vi "CTR_webSocketConfig_XML-JSON.vi"(8 "error in":errorcluster, 10 "webSocketCluster_typeDef in":T2, 11 "DOM document in":refnum<k20>) -> (0 "error out":errorcluster={"status"=TRUE, "code"=0, "source"=""}, 2 "webSocketCluster_typeDef out":T2, 3 "DOM document out":refnum<k20>)   [LabVIEW 2024]
uses:
  10f0a1c7-9ed0-4649-ba5a-dd6b15093da3.vi
  0a0fd023-9856-4cf8-bcff-a165bffb7d59.vi
  <vilib>/xml/Close Reference(Node).vi
  <vilib>/Utility/error.llb/Error Cluster From Error Code.vi
  <vilib>/ErrorRing/Error Ring.xnode
  <vilib>/Comparison/Less/Less Functor/Less Functor.lvclass
  <vilib>/xml/NI_XML.lvlib
  Control/webSocketCluster_typeDef.ctl
  Control/webSocketJsonConfig.ctl
panel:
  in  "webSocketJsonConfig":T1={"controls"=[{"channels"=[{"refDes"="OT-01", "role"="sensor", "units"="Deg F"}], "type"="temperature", "description"="LOX Tank Temperature 0%", "refDes"="OT-01", "subType"="", "details"={"absolute"=FALSE, "absoluteSensorRefDes"="NPT-01", "senseRefDes"="NPT-02"}}], "type"="config"}
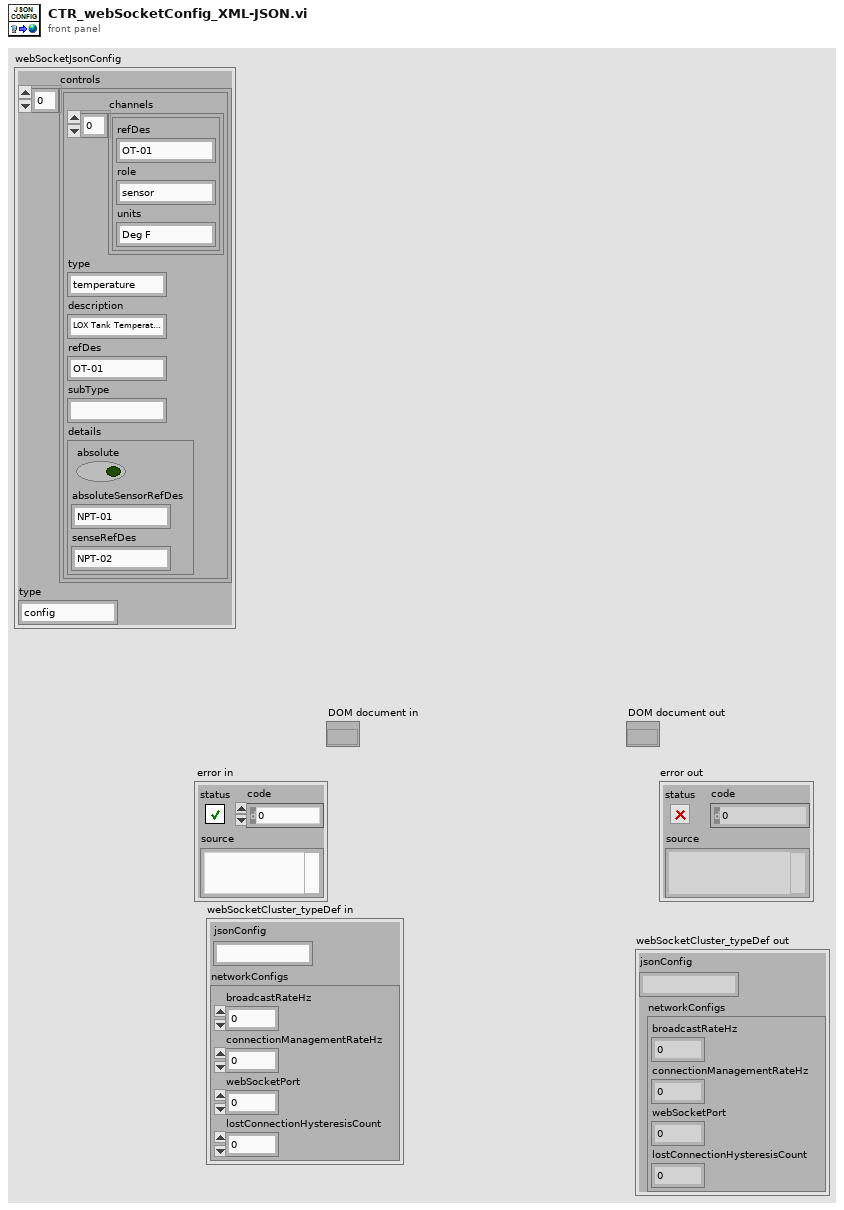
[diagram p1: front panel]
types:
  T1 = typedef "webSocketJsonConfig.ctl" = cluster{"controls":cluster{"channels":cluster{"refDes":string, "role":string, "units":string}[], "type":string, "description":string, "refDes":string, "subType":string, "details":cluster{"absolute":bool, "absoluteSensorRefDes":string, "senseRefDes":string}}[], "type":string}
  T2 = typedef "webSocketCluster_typeDef.ctl" = cluster{"networkConfigs":cluster{"broadcastRateHz":i32, "connectionManagementRateHz":i32, "webSocketPort":i32, "lostConnectionHysteresisCount":i32}, "jsonConfig":string}
  T3 = cluster{"channels":cluster{"refDes":string, "role":string, "units":string}[], "type":string, "description":string, "refDes":string, "subType":string, "details":cluster{"absolute":bool, "absoluteSensorRefDes":string, "senseRefDes":string}}[]
  T4 = cluster{"refDes":string, "role":string, "units":string}[]
  T5 = cluster{"absolute":bool, "absoluteSensorRefDes":string, "senseRefDes":string}
  T6 = cluster{"[0]":string, "[1]":string, "[2]":string}
  T7 = cluster{"refDes":string, "role":string, "units":string}
  T8 = cluster{"[0]":string, "[1]":string, "[2]":string, "[3]":string}
  T9 = cluster{"channels":cluster{"refDes":string, "role":string, "units":string}[], "type":string, "description":string, "refDes":string, "subType":string, "details":cluster{"absolute":bool, "absoluteSensorRefDes":string, "senseRefDes":string}}
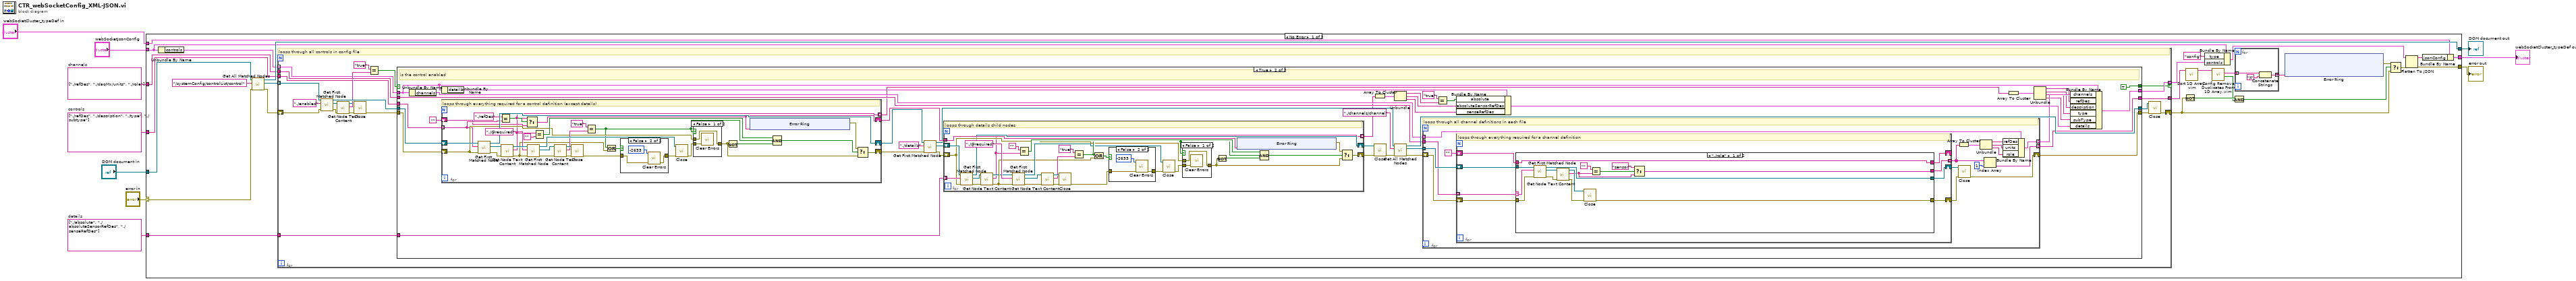
[diagram p0: block diagram]
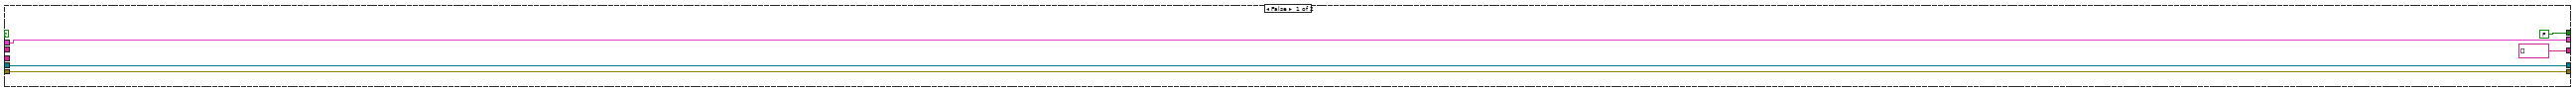
[diagram p2: hidden frame]
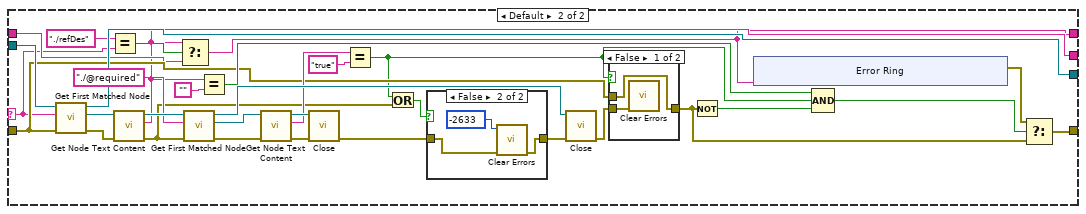
[diagram p7: hidden frame]
diagram:
  w1 = string[] ["./absolute", "./absoluteSensorRefDes", "./senseRefDes"]  # details
  w2 = string[] ["./refDes", "./description", "./type", "./subtype"]  # controls
  w7 = string[] ["./refDes", "./daqMx/units", "./role"]  # channels
  n1 = case shown="No Error" "error in" {
    selector: "error in" -> [w37 w297]
    tunnel: [w18 w297] -> w9
    tunnel: [w33 w296] -> w8
    tunnel: "DOM document in" -> [w38 w296]
    tunnel: w7 -> [w32 _]
    tunnel: "webSocketCluster_typeDef in" -> [w22 w295]
    tunnel: [w21 w295] -> w4
    tunnel: "webSocketJsonConfig" -> [w14 _]
    tunnel: w2 -> [w12 _]
    tunnel: w1 -> [w11 _]
    frame No Error {
      n2 = Unbundle By Name(w14) -> ("controls"=w13:T3)
      n3 = call <vilib>:"Get All Matched Nodes.vi"("error in (no error)"=w37, "XPath expression"="/systemConfig/controlList/control", "node in"=w38) -> ("error out"=w34:errorcluster, "node result array"=w35:refnum<k20>[], "node out"=w33:refnum<k20>)  [unwired: 6 in]
      n4 = for {
        tunnel: w35 -> [w61] mode=indexing
        shift-right: [w68] -> w28
        shift-left: w34 -> [w64]
        tunnel: w32 -> [w67]
        tunnel: [w54] -> w31 mode=concatenating
        tunnel: [w53] -> w17 mode=indexing if=w51
        tunnel: w13 -> [w52] mode=indexing
        tunnel: w12 -> [w50]
        tunnel: w11 -> [w49]
        # "loops through all controls in config file"
        n5 = call <vilib>:"Get First Matched Node.vi"("error in (no error)"=w64, "XPath expression"="./enabled", "node in"=w61) -> ("error out"=w65:errorcluster, "node result"=w59:refnum<k20>, "node out"=w62:refnum<k20>)  [unwired: 6 in]
        n6 = call <vilib>:"Get Node Text Content.vi"("error in (no error)"=w65, "node in"=w59) -> ("error out"=w66:errorcluster, "node text"=w57:string, "node out"=w56:refnum<k20>)  [unwired: 7 in]
        n7 = call-poly <vilib>:"Close.vi"("error in (no error)"=w66, "node"=w56) -> ("error out"=w63:errorcluster)  [unwired: 7 in]
        n8 = Equal?(x="true", y=w57) -> (x = y?=w58:bool)
        n9 = case shown="True" w58 {
          tunnel: w63 -> [w74 w106]
          tunnel: w62 -> [w75 w105]
          tunnel: [w74 w114] -> w70
          tunnel: [w75 w113] -> w69
          tunnel: w67 -> [_ w103]
          tunnel: [string[] [] w112] -> w54
          tunnel: [w71 w111] -> w53
          tunnel: w52 -> [w71 w85]
          tunnel: [FALSE TRUE] -> w51
          tunnel: w50 -> [_ w104]
          tunnel: w49 -> [_ w96]
          frame False {
          }
          frame True {
            # "is the control enabled"
            n10 = Unbundle By Name(w85) -> ("channels"=w108:T4)
            n11 = Unbundle By Name(w85) -> ("details"=w84:T5)
            n12 = for {
              shift-right: [w191] -> w91
              shift-left: w105 -> [w194]
              tunnel: w104 -> [w166] mode=indexing
              shift-right: [w176] -> w94
              shift-left: w106 -> [w172]
              tunnel: [w163] -> w102 mode=indexing
              shift-right: [w162] -> w95
              shift-left: "" -> [w164]
              # "loops through everything required for a control definition (except details)"
              n13 = call <vilib>:"Get First Matched Node.vi"("error in (no error)"=w172, "XPath expression"=w166, "node in"=w194) -> ("error out"=w193:errorcluster, "node result"=w192:refnum<k20>, "node out"=w191:refnum<k20>)  [unwired: 6 in]
              n14 = Equal?(x="./refDes", y=w166) -> (x = y?=w165:bool)
              n15 = call <vilib>:"Get Node Text Content.vi"("error in (no error)"=w193, "node in"=w192) -> ("error out"=w168:errorcluster, "node text"=w163:string, "node out"=w190:refnum<k20>)  [unwired: 7 in]
              n16 = Select(t=w163, s=w165, f=w164) -> (s? t:f=w162:string)
              n17 = call <vilib>:"Get First Matched Node.vi"("error in (no error)"=w168, "XPath expression"="./@required" ("string"), "node in"=w190) -> ("error out"=w189:errorcluster, "node result"=w188:refnum<k20>, "node out"=w187:refnum<k20>)  [unwired: 6 in]
              n18 = Equal?(x=w163, y="") -> (x = y?=w180:bool)
              n19 = call <vilib>:"Get Node Text Content.vi"("error in (no error)"=w189, "node in"=w188) -> ("error out"=w186:errorcluster, "node text"=w183:string, "node out"=w185:refnum<k20>)  [unwired: 7 in]
              n20 = call-poly <vilib>:"Close.vi"("error in (no error)"=w186, "node"=w185) -> ("error out"=w174:errorcluster)  [unwired: 7 in]
              n21 = Equal?(x="true" ("y"), y=w183) -> (x = y?=w169:bool)
              n22 = Or(x=w169, y=w168) -> (x .or. y?=w170:bool)
              n23 = case shown="False" w170 {
                tunnel: [w198 w200] -> w175
                tunnel: w174 -> [w198 w199]
                frame True {
                }
                frame False {
                  n24 = call <vilib>:"Clear Errors.vi"("error in (no error)"=w199, "specific error code to clear (0: all)"=-2633) -> ("error out"=w200:errorcluster)  [unwired: 4 in, 1 out]
                }
              }
              n25 = call-poly <vilib>:"Close.vi"("error in (no error)"=w175, "node"=w187) -> ("error out"=w173:errorcluster)  [unwired: 7 in]
              n26 = case shown="False" w169 {
                tunnel: w173 -> [w196 w197]
                tunnel: w172 -> [w195 _]
                tunnel: [w195 w197] -> w171
                frame False {
                  n27 = call <vilib>:"Clear Errors.vi"("error in (no error)"=w196) -> ()  [unwired: 5 in, 2 out]
                }
                frame True {
                }
              }
              n28 = Not(x=w171) -> (.not. x?=w179:bool)
              n29 = xnode "Error Ring"("parameter 0"=w162) -> ("error out"=w177:errorcluster)
              n30 = Compound Arithmetic op=AND(w180, w169, w179) -> (w178:bool)
              n31 = Select(t=w177, s=w178, f=w171) -> (s? t:f=w176:errorcluster)
            }
            n32 = call <vilib>:"Get First Matched Node.vi"("error in (no error)"=w94, "XPath expression"="./details", "node in"=w91) -> ("error out"=w93:errorcluster, "node result"=w89:refnum<k20>, "node out"=w90:refnum<k20>)  [unwired: 6 in]
            n33 = for {
              shift-right: [w144] -> w88
              shift-left: w93 -> [w122]
              tunnel: w96 -> [w123] mode=indexing
              tunnel: w95 -> [w143]
              shift-right: [w120] -> w87
              shift-left: w89 -> [w124]
              tunnel: [w118] -> w81 mode=indexing
              # "loops through details child nodes"
              n34 = call <vilib>:"Get First Matched Node.vi"("error in (no error)"=w122, "XPath expression"=w123, "node in"=w124) -> ("error out"=w125:errorcluster, "node result"=w126:refnum<k20>, "node out"=w120:refnum<k20>)  [unwired: 6 in]
              n35 = call <vilib>:"Get Node Text Content.vi"("error in (no error)"=w125, "node in"=w126) -> ("error out"=w121:errorcluster, "node text"=w118:string, "node out"=w119:refnum<k20>)  [unwired: 7 in]
              n36 = call <vilib>:"Get First Matched Node.vi"("error in (no error)"=w121, "XPath expression"="./@required" ("string"), "node in"=w119) -> ("error out"=w134:errorcluster, "node result"=w133:refnum<k20>, "node out"=w129:refnum<k20>)  [unwired: 6 in]
              n37 = Equal?(x="", y=w118) -> (x = y?=w138:bool)
              n38 = call <vilib>:"Get Node Text Content.vi"("error in (no error)"=w134, "node in"=w133) -> ("error out"=w132:errorcluster, "node text"=w128:string, "node out"=w131:refnum<k20>)  [unwired: 7 in]
              n39 = call-poly <vilib>:"Close.vi"("error in (no error)"=w132, "node"=w131) -> ("error out"=w130:errorcluster)  [unwired: 7 in]
              n40 = Equal?(x="true", y=w128) -> (x = y?=w135:bool)
              n41 = Or(x=w135, y=w121) -> (x .or. y?=w140:bool)
              n42 = case shown="False" w140 {
                tunnel: [w151 w153] -> w142
                tunnel: w130 -> [w151 w152]
                frame True {
                }
                frame False {
                  n43 = call <vilib>:"Clear Errors.vi"("error in (no error)"=w152, "specific error code to clear (0: all)"=-2633) -> ("error out"=w153:errorcluster)  [unwired: 4 in, 1 out]
                }
              }
              n44 = call-poly <vilib>:"Close.vi"("error in (no error)"=w142, "node"=w129) -> ("error out"=w141:errorcluster)  [unwired: 7 in]
              n45 = case shown="False" w135 {
                tunnel: w141 -> [w149 w150]
                tunnel: w122 -> [w148 _]
                tunnel: [w148 w150] -> w139
                frame False {
                  n46 = call <vilib>:"Clear Errors.vi"("error in (no error)"=w149) -> ()  [unwired: 5 in, 2 out]
                }
                frame True {
                }
              }
              n47 = Not(x=w139) -> (.not. x?=w145:bool)
              n48 = xnode "Error Ring"("parameter 0"=w143) -> ("error out"=w147:errorcluster)
              n49 = Compound Arithmetic op=AND(w138, w135, w145) -> (w146:bool)
              n50 = Select(t=w147, s=w146, f=w139) -> (s? t:f=w144:errorcluster)
            }
            n51 = Array To Cluster(array=w81) -> (cluster=w82:T6)
            n52 = call-poly <vilib>:"Close.vi"("error in (no error)"=w88, "node"=w87) -> ("error out"=w86:errorcluster)  [unwired: 7 in]
            n53 = Unbundle(w82) -> ("[0]"=w78:string, "[1]"=w79:string, "[2]"=w80:string)
            n54 = call <vilib>:"Get All Matched Nodes.vi"("error in (no error)"=w86, "XPath expression"="./channels/channel", "node in"=w90) -> ("error out"=w116:errorcluster, "node result array"=w115:refnum<k20>[], "node out"=w113:refnum<k20>)  [unwired: 6 in]
            n55 = for {
              shift-right: [w222] -> w114
              shift-left: w116 -> [w223]
              tunnel: w115 -> [w224] mode=indexing
              tunnel: w103 -> [w221]
              tunnel: [w218] -> w112 mode=indexing
              tunnel: [w216] -> w109 mode=indexing
              tunnel: w108 -> [w217] mode=indexing
              # "loops through all channel definitions in each file"
              n56 = for {
                shift-right: [w231] -> w215
                shift-left: w224 -> [w232]
                tunnel: w221 -> [w225] mode=indexing
                shift-right: [w230] -> w214
                shift-left: w223 -> [w229]
                tunnel: [w227] -> w212 mode=indexing
                shift-right: [w226] -> _
                shift-left: "" -> [w228]
                # "loops through everything required for a channel definition"
                n57 = case shown="\"./role\"" w225 {
                  selector: w225 -> [w243 w248]
                  tunnel: w232 -> [w242 w280]
                  tunnel: [w241 w277] -> w231
                  tunnel: [w238 w262] -> w230
                  tunnel: w229 -> [w244 w258]
                  tunnel: w228 -> [w247 w251]
                  tunnel: [w233 w250] -> w227
                  tunnel: [w247 w249] -> w226
                  frame "./role" {
                    n58 = call <vilib>:"Get First Matched Node.vi"("error in (no error)"=w244, "XPath expression"=w243, "node in"=w242) -> ("error out"=w246:errorcluster, "node result"=w240:refnum<k20>, "node out"=w241:refnum<k20>)  [unwired: 6 in]
                    n59 = call <vilib>:"Get Node Text Content.vi"("error in (no error)"=w246, "node in"=w240) -> ("error out"=w245:errorcluster, "node text"=w234:string, "node out"=w239:refnum<k20>)  [unwired: 7 in]
                    n60 = call-poly <vilib>:"Close.vi"("error in (no error)"=w245, "node"=w239) -> ("error out"=w238:errorcluster)  [unwired: 7 in]
                    n61 = Equal?(x="", y=w234) -> (x = y?=w236:bool)
                    n62 = Select(t="sensor", s=w236, f=w234) -> (s? t:f=w233:string)
                  }
                  frame Default {
                    n63 = call <vilib>:"Get First Matched Node.vi"("error in (no error)"=w258, "XPath expression"=w248, "node in"=w280) -> ("error out"=w279:errorcluster, "node result"=w278:refnum<k20>, "node out"=w277:refnum<k20>)  [unwired: 6 in]
                    n64 = Equal?(x="./refDes", y=w248) -> (x = y?=w252:bool)
                    n65 = call <vilib>:"Get Node Text Content.vi"("error in (no error)"=w279, "node in"=w278) -> ("error out"=w254:errorcluster, "node text"=w250:string, "node out"=w276:refnum<k20>)  [unwired: 7 in]
                    n66 = Select(t=w250, s=w252, f=w251) -> (s? t:f=w249:string)
                    n67 = call <vilib>:"Get First Matched Node.vi"("error in (no error)"=w254, "XPath expression"="./@required" ("string"), "node in"=w276) -> ("error out"=w275:errorcluster, "node result"=w274:refnum<k20>, "node out"=w273:refnum<k20>)  [unwired: 6 in]
                    n68 = Equal?(x=w250, y="") -> (x = y?=w266:bool)
                    n69 = call <vilib>:"Get Node Text Content.vi"("error in (no error)"=w275, "node in"=w274) -> ("error out"=w272:errorcluster, "node text"=w269:string, "node out"=w271:refnum<k20>)  [unwired: 7 in]
                    n70 = call-poly <vilib>:"Close.vi"("error in (no error)"=w272, "node"=w271) -> ("error out"=w260:errorcluster)  [unwired: 7 in]
                    n71 = Equal?(x=w269, y="true") -> (x = y?=w255:bool)
                    n72 = Or(x=w255, y=w254) -> (x .or. y?=w256:bool)
                    n73 = case shown="False" w256 {
                      tunnel: [w291 w293] -> w261
                      tunnel: w260 -> [w291 w292]
                      frame True {
                      }
                      frame False {
                        n74 = call <vilib>:"Clear Errors.vi"("error in (no error)"=w292, "specific error code to clear (0: all)"=-2633) -> ("error out"=w293:errorcluster)  [unwired: 4 in, 1 out]
                      }
                    }
                    n75 = call-poly <vilib>:"Close.vi"("error in (no error)"=w261, "node"=w273) -> ("error out"=w259:errorcluster)  [unwired: 7 in]
                    n76 = case shown="False" w255 {
                      tunnel: w259 -> [w282 w283]
                      tunnel: w258 -> [w281 _]
                      tunnel: [w281 w283] -> w257
                      frame False {
                        n77 = call <vilib>:"Clear Errors.vi"("error in (no error)"=w282) -> ()  [unwired: 5 in, 2 out]
                      }
                      frame True {
                      }
                    }
                    n78 = Not(x=w257) -> (.not. x?=w265:bool)
                    n79 = xnode "Error Ring"("parameter 0"=w249) -> ("error out"=w263:errorcluster)
                    n80 = Compound Arithmetic op=AND(w266, w255, w265) -> (w264:bool)
                    n81 = Select(t=w263, s=w264, f=w257) -> (s? t:f=w262:errorcluster)
                  }
                }
              }
              n82 = Array To Cluster(array=w212) -> (cluster=w213:T6)
              n83 = call-poly <vilib>:"Close.vi"("error in (no error)"=w214, "node"=w215) -> ("error out"=w222:errorcluster)  [unwired: 7 in]
              n84 = Unbundle(w213) -> ("[0]"=w211:string, "[1]"=w210:string, "[2]"=w209:string)
              n85 = Index Array(array=w212, index=1) -> (element=w218:string)
              n86 = Bundle By Name(cluster=w217, "refDes"=w211, "units"=w210, "role"=w209) -> (w216:T7)
            }
            n87 = Equal?(x="true", y=w78) -> (x = y?=w76:bool)
            n88 = Bundle By Name(cluster=w84, "absolute"=w76, "absoluteSensorRefDes"=w79, "senseRefDes"=w80) -> (w83:T5)
            n89 = Array To Cluster(array=w102) -> (cluster=w101:T8)
            n90 = Unbundle(w101) -> ("[0]"=w100:string, "[1]"=w99:string, "[2]"=w98:string, "[3]"=w97:string)
            n91 = Bundle By Name(cluster=w85, "channels"=w109, "refDes"=w100, "description"=w99, "type"=w98, "subType"=w97, "details"=w83) -> (w111:T9)
          }
        }
        n92 = call-poly <vilib>:"Close.vi"("error in (no error)"=w70, "node"=w69) -> ("error out"=w68:errorcluster)  [unwired: 7 in]
      }
      n93 = Not(x=w28) -> (.not. x?=w29:bool)
      n94 = call "Sort 1D Array.vim"("unsorted array"=w31) -> ("sorted array"=w25:string[])  [unwired: 10 in]
      n95 = Bundle By Name(cluster=w14, "type"="config", "controls"=w17) -> (w15:T1)
      n96 = call "Config Remove Duplicates From 1D Array.vim"("array"=w25) -> ("duplicates?"=w24:bool, "array of duplicates"=w23:string[])  [unwired: 8 in, 1 out]
      n97 = And(x=w29, y=w24) -> (x .and. y?=w30:bool)
      n98 = for {
        tunnel: w23 -> [w41] mode=indexing
        tunnel: [w39] -> w26 mode=concatenating
        n99 = Concatenate Strings(w41, "\t") -> (w39:string)
      }
      n100 = xnode "Error Ring"("parameter 0"=w26) -> ("error out"=w27:errorcluster)
      n101 = Select(t=w27, s=w30, f=w28) -> (s? t:f=w19:errorcluster)
      n102 = Flatten To JSON(anything=w15, error in (no error)=w19) -> (JSON string=w20:string, 11:w18:errorcluster)  [unwired: 1 in]
      n103 = Bundle By Name(cluster=w22, "jsonConfig"=w20) -> (w21:T2)
    }
    frame Error {
    }
  }
  "error out" <- w9
  "DOM document out" <- w8
  "webSocketCluster_typeDef out" <- w4
